vi "AddDropletDetectionOverlay2Image.vi"(6 "Circles (Calibrated)":T2(array[cluster]) {"Position"."Y" format="%.2f"; "Position"."X" format="%.2f"}, 8 "error in (no error)":errorcluster, 9 "Mag":T1=enum."20x_LM", 10 "Matches (pixel)":T3(array[cluster]), 11 "Input Image":T4) -> (0 "error out":errorcluster, 3 "Output Image":T4)   [LabVIEW 2013]
doc: "Use this template to build a VI to use as a subVI."
uses:
  <vilib>/vision/Image Controls.llb/IMAQ Image.ctl
  Mag.ctl
  <vilib>/Analysis/NI_AALBase.lvlib
panel:
  out "Reference Image":T4(plugin-control)
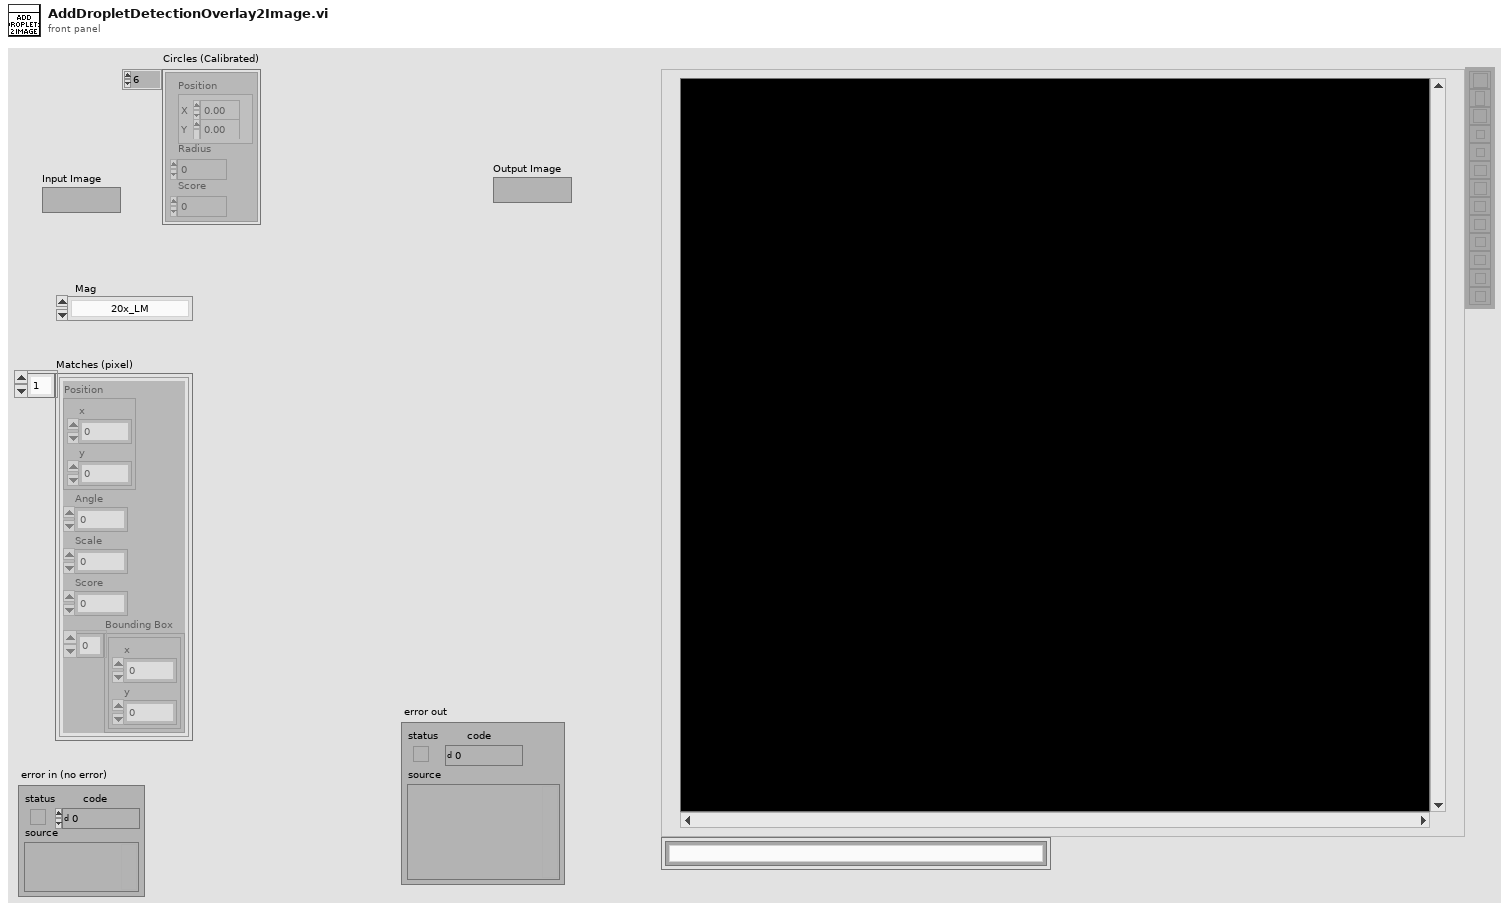
[diagram p1: front panel]
types:
  T1 = typedef "Mag.ctl" = enum16{"10x_LM", "20x_LM", "50x_S", "100x_im"}
  T2 = cluster{"Position":cluster{"X":sgl, "Y":sgl}, "Radius":dbl, "Score":dbl}[]
  T3 = cluster{"Position":cluster{"x":sgl, "y":sgl}, "Angle":sgl, "Scale":sgl, "Score":sgl, "Bounding Box":cluster{"x":sgl, "y":sgl}[]}[]
  T4 = typedef "IMAQ Image.ctl" = refnum<image>
  T5 = cluster{"Desired Font (Application)":enum16{"User-specified Font", "Application Font", "System Font", "Dialog Font"}, "[User-specified Font]":cluster{"Font Name":string, "Size":i16, "Strikeout?":bool, "Italic?":bool, "Underline?":bool, "Outline?":bool, "Shadow?":bool, "Bold?":bool, "Rotation Angle":dbl}, "Horizontal Alignment":i16, "Vertical Alignment":i16}
  T6 = cluster{"Array[0]":i32, "Array[1]":i32, "Array[2]":i32, "Array[3]":i32}
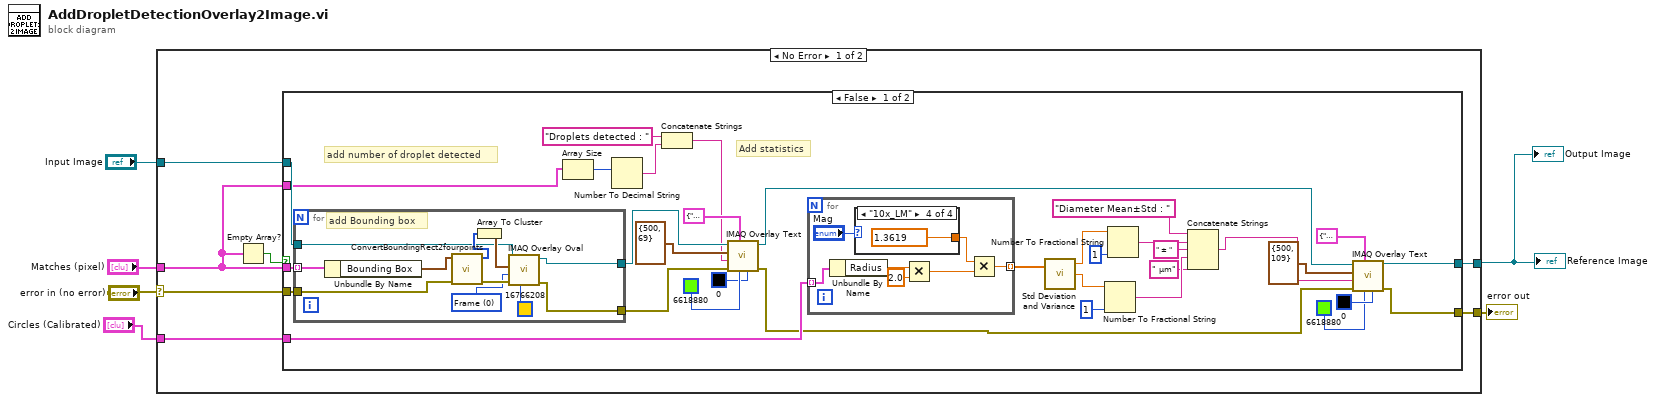
[diagram p0: block diagram]
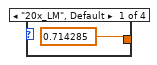
[diagram p2: hidden frame]
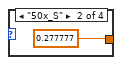
[diagram p3: hidden frame]
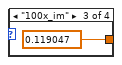
[diagram p4: hidden frame]
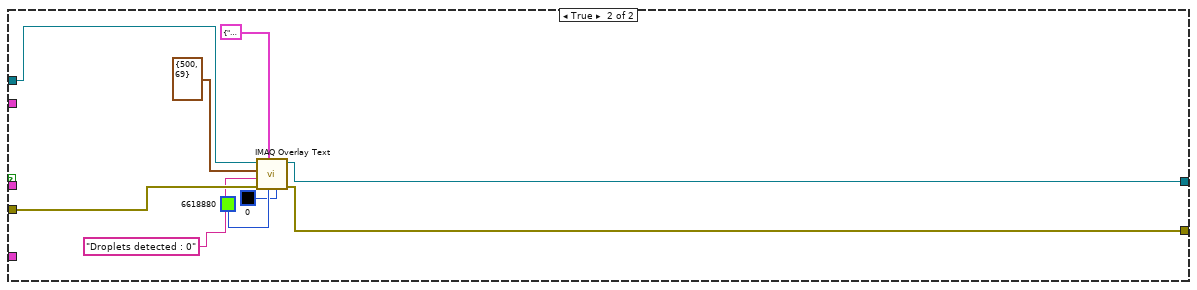
[diagram p5: hidden frame]
diagram:
  n1 = case shown="No Error" "error in (no error)" {
    selector: "error in (no error)" -> [w13 w80]
    tunnel: [w10 w80] -> w5
    tunnel: "Input Image" -> [w12 w79]
    tunnel: [w11 w79] -> w3
    tunnel: "Matches (pixel)" -> [w8 _]
    tunnel: "Circles (Calibrated)" -> [w7 _]
    frame No Error {
      n2 = Empty Array?(array=w8) -> (empty?=w9:bool)
      n3 = case shown="False" w9 {
        tunnel: w13 -> [w47 w73]
        tunnel: w12 -> [w46 w75]
        tunnel: [w28 w74] -> w11
        tunnel: [w27 w72] -> w10
        tunnel: w8 -> [w45 _]
        tunnel: w8 -> [w39 _]
        tunnel: w7 -> [w36 _]
        frame False {
          # "Add statistics"
          # "add number of droplet detected"
          n4 = for {
            tunnel: w45 -> [w69] mode=indexing
            tunnel: w47 -> [w67]
            tunnel: w46 -> [w63]
            tunnel: [w62] -> w41
            tunnel: [w61] -> w40
            w60 = u32 0 items=["Frame", "Fill", "Highlight"] ("Drawing Mode (Frame)")
            # "add Bounding box"
            n5 = Unbundle By Name(w69) -> ("Bounding Box"=w68:cluster{"x":sgl, "y":sgl}[])
            n6 = call "ConvertBoundingRect2fourpoints.vi"("Error In"=w67, "Bounding Box"=w68) -> ("Error Out"=w64:errorcluster, "Array"=w65:i32[])  [unwired: 8 in]
            n7 = Array To Cluster(array=w65) -> (cluster=w66:T6)
            n8 = call "IMAQ Overlay Oval"("Color"=u32 16766208, "error in (no error)"=w64, "Drawing Mode (Frame)"=w60, "Bounding Rectangle"=w66, "Image"=w63) -> ("error out"=w61:errorcluster, "Image Out"=w62:T4)  [unwired: 5 in]
          }
          n9 = Array Size(array=w39) -> (size(s)=w38:i32)
          n10 = Number To Decimal String(number=w38) -> (decimal integer string=w15:string)  [unwired: 1 in]
          n11 = Concatenate Strings("Droplets detected : " ("string"), w15) -> (w14:string)
          n12 = call "IMAQ Overlay Text"("BG Color (Transparent)"=u32 0, "Text Color (black)"=u32 6618880, "Font, Size & Style"=T5 {"Desired Font (Application)"=enum."User-specified Font", "[User-specified Font]"={"Font Name"="", "Size"=32, "Strikeout?"=FALSE, "Italic?"=FALSE, "Underline?"=FALSE, "Outline?"=FALSE, "Shadow?"=FALSE, "Bold?"=TRUE, "Rotation Angle"=0.0}, "Horizontal Alignment"=2, "Vertical Alignment"=2}, "error in (no error)"=w40, "String"=w14, "Origin"=cluster{"X":i32, "Y":i32} {"X"=500, "Y"=69}, "Image"=w41) -> ("error out"=w30:errorcluster, "Image Out"=w29:T4)  [unwired: 3 in]
          n13 = for {
            tunnel: w36 -> [w54] mode=indexing
            tunnel: [w48] -> w35 mode=indexing
            n14 = Unbundle By Name(w54) -> ("Radius"=w53:dbl)
            n15 = case shown="\"10x_LM\"" "Mag" {
              tunnel: [w55 w56 w57 w58] -> w50
              frame "20x_LM", Default {
                w55 = 0.714285 items=["5x_M_BD"=2.731524, "10x_M"=1.3634, "10xM_BD"=1.3543, "10x_ph1"=1.3439, "20x_S"=0.68129, "20x_LM"=0.714285, "50x_S"=0.277777, "100x_im"=0.119047] ("Magnification (Microns/Pixel)")
              }
              frame "50x_S" {
                w56 = 0.277777 items=["5x_M_BD"=2.731524, "10x_M"=1.3634, "10xM_BD"=1.3543, "10x_ph1"=1.3439, "20x_S"=0.68129, "20x_LM"=0.714285, "50x_S"=0.277777, "100x_im"=0.119047] ("Magnification (Microns/Pixel)")
              }
              frame "100x_im" {
                w57 = 0.119047 items=["5x_M_BD"=2.731524, "10x_M"=1.3634, "10xM_BD"=1.3543, "10x_ph1"=1.3439, "20x_S"=0.68129, "20x_LM"=0.714285, "50x_S"=0.277777, "100x_im"=0.119047] ("Magnification (Microns/Pixel)")
              }
              frame "10x_LM" {
                w58 = 1.3619 items=["10x_LM"=1.3619, "5x_M_BD"=2.731524, "10x_M"=1.3634, "10xM_BD"=1.3543, "10x_ph1"=1.3439, "20x_S"=0.68129, "20x_LM"=0.714285, "50x_S"=0.277777, "100x_im"=0.119047] ("Magnification (Microns/Pixel)")
              }
            }
            n16 = Multiply(x=w53, y=2.0) -> (x*y=w49:dbl)
            n17 = Multiply(x=w50, y=w49) -> (x*y=w48:dbl)
          }
          n18 = call <vilib>:"Std Deviation and Variance.vi"("X"=w35) -> ("mean"=w24:dbl, "standard deviation"=w23:dbl)  [unwired: 1 in, 1 out]
          n19 = Number To Fractional String(number=w23, precision (6)=i16 1) -> (F-format string=w19:string)  [unwired: 2 in]
          n20 = Number To Fractional String(number=w24, precision (6)=i16 1) -> (F-format string=w21:string)  [unwired: 2 in]
          n21 = Concatenate Strings("Diameter Mean±Std : " ("string"), w21, " ± " ("string"), w19, " µm" ("string")) -> (w18:string)
          n22 = call "IMAQ Overlay Text"("BG Color (Transparent)"=u32 0, "Text Color (black)"=u32 6618880, "Font, Size & Style"=T5 {"Desired Font (Application)"=enum."User-specified Font", "[User-specified Font]"={"Font Name"="", "Size"=32, "Strikeout?"=FALSE, "Italic?"=FALSE, "Underline?"=FALSE, "Outline?"=FALSE, "Shadow?"=FALSE, "Bold?"=TRUE, "Rotation Angle"=0.0}, "Horizontal Alignment"=2, "Vertical Alignment"=2}, "error in (no error)"=w30, "String"=w18, "Origin"=cluster{"X":i32, "Y":i32} {"X"=500, "Y"=109}, "Image"=w29) -> ("error out"=w27:errorcluster, "Image Out"=w28:T4)  [unwired: 3 in]
        }
        frame True {
          n23 = call "IMAQ Overlay Text"("BG Color (Transparent)"=u32 0, "Text Color (black)"=u32 6618880, "Font, Size & Style"=T5 {"Desired Font (Application)"=enum."User-specified Font", "[User-specified Font]"={"Font Name"="", "Size"=32, "Strikeout?"=FALSE, "Italic?"=FALSE, "Underline?"=FALSE, "Outline?"=FALSE, "Shadow?"=FALSE, "Bold?"=TRUE, "Rotation Angle"=0.0}, "Horizontal Alignment"=2, "Vertical Alignment"=2}, "error in (no error)"=w73, "String"="Droplets detected : 0" ("string"), "Origin"=cluster{"X":i32, "Y":i32} {"X"=500, "Y"=69}, "Image"=w75) -> ("error out"=w72:errorcluster, "Image Out"=w74:T4)  [unwired: 3 in]
        }
      }
    }
    frame Error {
    }
  }
  "error out" <- w5
  "Reference Image" <- w3
  "Output Image" <- w3
